vi "Stage_z_stack.vi"(0 "SPIIPLUSCOM660Lib.IAsyncChannel IN":refnum<k7>, 5 "Number of slices":dbl, 7 "Z step size (um)":dbl, 9 "delay between steps (ms)":dbl, 11 "error IN":errorcluster) -> (4 "SPIIPLUSCOM660Lib.IAsyncChannel OUT":refnum<k7>, 15 "error OUT":errorcluster)   [LabVIEW 2020]
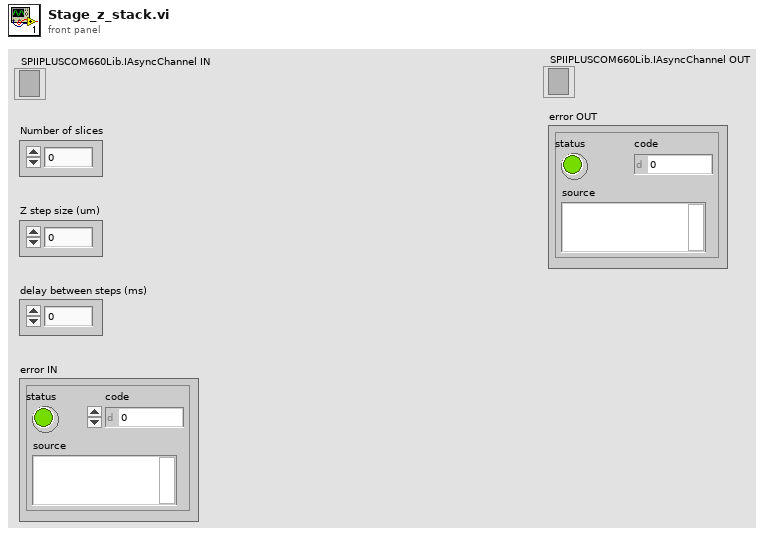
[diagram p1: front panel]
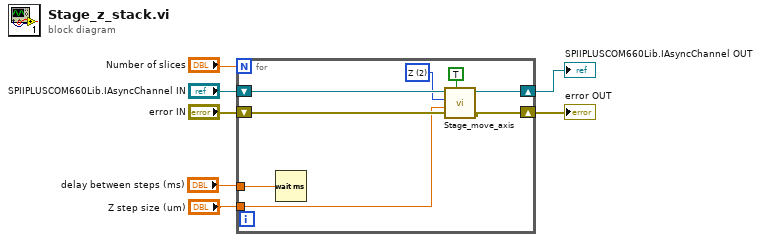
[diagram p0: block diagram]
diagram:
  n1 = for {
    N: "Number of slices" -> [_]
    tunnel: "Z step size (um)" -> [w9]
    shift-right: [w12] -> w5
    shift-left: "SPIIPLUSCOM660Lib.IAsyncChannel IN" -> [w14]
    shift-right: [w11] -> w4
    shift-left: "error IN" -> [w13]
    tunnel: "delay between steps (ms)" -> [w15]
    w10 = u16 2 items=["X", "Y", "Z"] ("Axes Select")
    n2 = Wait (ms)(milliseconds to wait=w15) -> ()  [unwired: 1 out]
    n3 = call "Stage_move_axis.vi"("Direction true means positive increment"=TRUE, "error in (no error)"=w13, "Distance micrometer"=w9, "Axes Select"=w10, "reference IN"=w14) -> ("error OUT"=w11:errorcluster, "reference OUT"=w12:refnum<k7>)  [unwired: 5 in]
  }
  "SPIIPLUSCOM660Lib.IAsyncChannel OUT" <- w5
  "error OUT" <- w4
